vi "Home.TestLauncher.vi"() -> ()   [LabVIEW 2022 SP3, in "Home.lvclass"]
uses:
  Home.lvclass
  Typedefs/Home State--enum.ctl
  <vilib>/JKI/JKI SMO/SMO/Typedefs/SMOState --Enum.ctl
  C:/Program Files (x86)/National Instruments/LabVIEW 2022/vi.lib/JKI/JKI SMO/SMO/SMO.lvclass
  <vilib>/JKI/JKI SMO/SMO/SMO.lvclass/SMO.ctl
  <vilib>/JKI/JKI SMO/SMO/Private/ReftoDVR--SMO.vi
  Home.lvclass/Home.ctl
  <vilib>/JKI/JKI SMO/SMO/SMO.lvclass
  D:/DSUsers/uib01493/000_SD_Card/009_Projects/CIS_580/SReTT_GUI/002_SRC/Home/Home.lvclass
panel:
  out "SMO State":T1
  in  "Embed?":bool=TRUE
  out "UI State":T2
  out "error out":errorcluster
  in  "Stop":bool
  # "SMO.UI_Embedded Test Launcher"
  # "For instructions on how to use the JKI State Machine Objects, examples and video tutorials, visit:\nhttp://jki.net/state-machine-objects/\n\nJKI State Machine Objects™\nhttp://jki.net/state-machine-objects/\nCopyright (C) 2005-2015, JKI <info@jki.net>\nALL RIGHTS RESERVED"
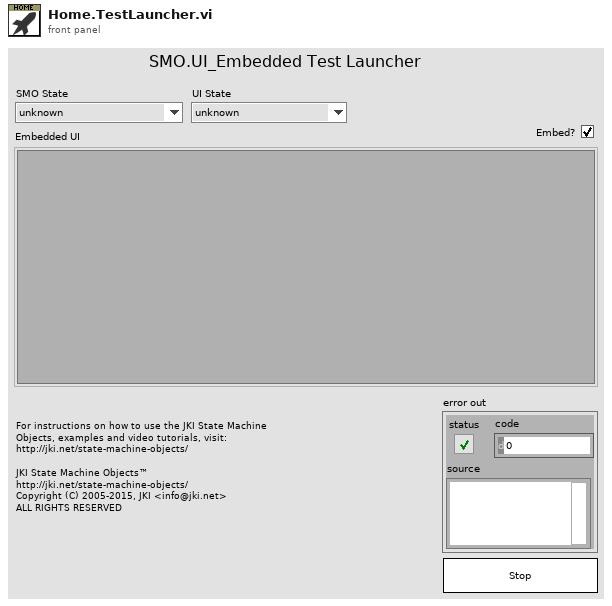
[diagram p1: front panel]
types:
  T1 = typedef "SMO.lvclass/SMOState --Enum.ctl" = enum16{"unknown", "Created", "Started", "Stopped"}
  T2 = typedef "Home.lvclass/Home State--enum.ctl" = enum16{"unknown", "Opened", "Embedded", "Closed"}
  T3 = typedef "SMO.lvclass/Public Events.ctl" = cluster{"Error":refnum<user-event>, "State":refnum<user-event>, "Reserve State":refnum<user-event>}
  T4 = typedef "Home.lvclass/PublicEvents--Cluster.ctl" = cluster{"UI State":refnum<user-event>}
  T5 = cluster{"Event Registration Refnum":refnum<event-registration>}
  T6 = typedef "Home.lvclass/SMO.UI_Embed State--enum.ctl" = enum16{"unknown", "Opened", "Embedded", "Closed"}
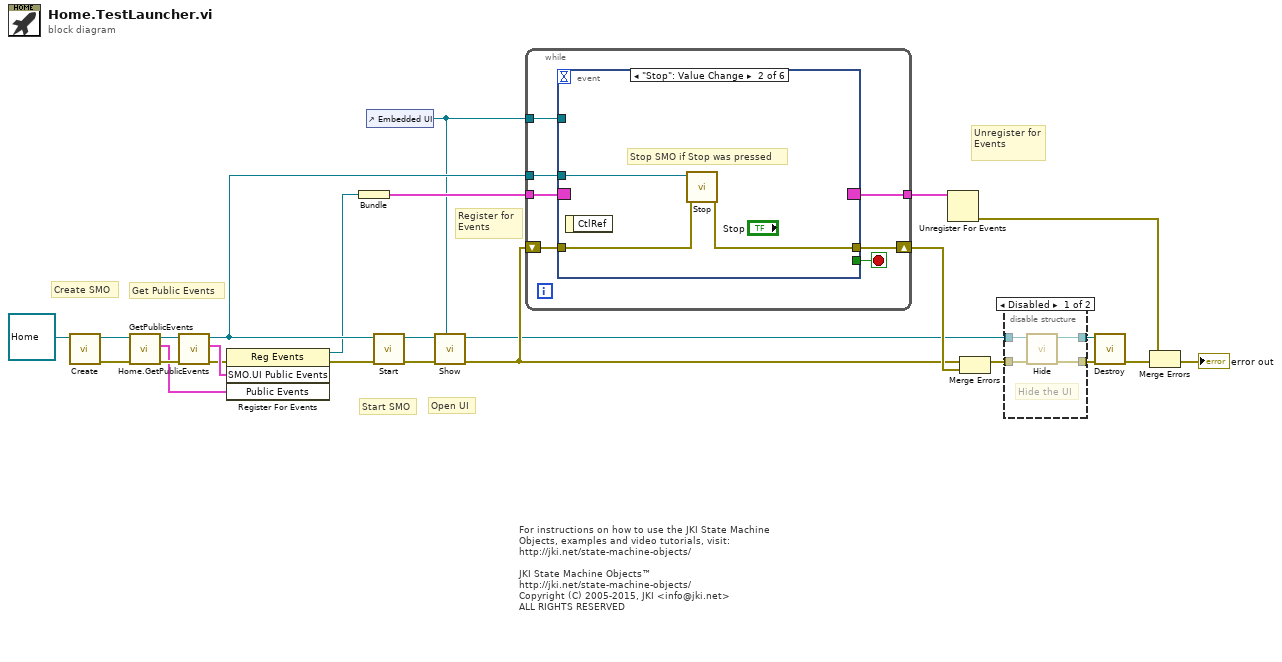
[diagram p0: block diagram]
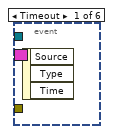
[diagram p3: hidden frame]
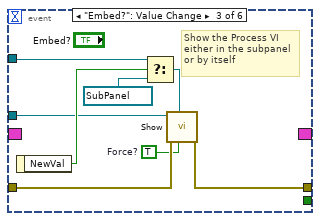
[diagram p4: hidden frame]
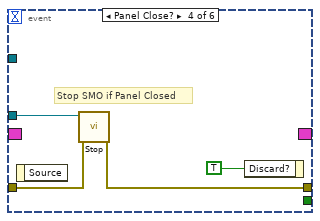
[diagram p5: hidden frame]
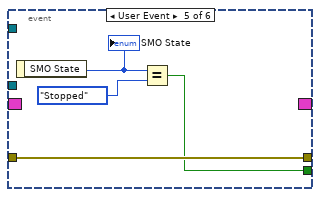
[diagram p6: hidden frame]
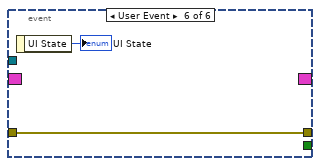
[diagram p7: hidden frame]
diagram:
  # "For instructions on how to use the JKI State Machine Objects, examples and video tutorials, visit:\nhttp://jki.net/state-machine-objects/\n\nJKI State Machine Objects™\nhttp://jki.net/state-machine-objects/\nCopyright (C) 2005-2015, JKI <info@jki.net>\nALL RIGHTS RESERVED"
  # "Get Public Events"
  # "Start SMO"
  # "Create SMO"
  # "Open UI"
  # "Unregister for Events"
  # "Register for Events"
  n1 = call <vilib>:"Create.vi"("SMO"=refnum<class "Home.lvclass"> refnum ("SMO.UI.lvclass")) -> ("error out"=w13:errorcluster, "SMO out"=w11:refnum<class "Home.lvclass">)  [unwired: 8 in, 1 out]
  n2 = call <vilib>:"GetPublicEvents.vi"("error in (no error)"=w13, "SMO"=w11) -> ("error out"=w12:errorcluster, "Public Events"=w9:T3, "SMO out"=w10:refnum<class "Home.lvclass">)  [unwired: 7 in]
  n3 = call "Home.GetPublicEvents.vi"("error in (no error)"=w12, "Home"=w10) -> ("error out"=w15:errorcluster, "SMO.UI Public Events"=w17:T4, "Home out"=w18:refnum<class "Home.lvclass">)  [unwired: 7 in]
  n4 = register-events(error in=w15, w17, w9) -> (reference out=w16:refnum<event-registration>, error out=w14:errorcluster)  [unwired: 1 in]
  n5 = Bundle("Event Registration Refnum"=w16) -> (w24:T5)  [unwired: 1 in]
  n6 = control-ref of="Embedded UI"() -> (w5:refnum<vi>)
  n7 = call <vilib>:"Start.vi"("error in (no error)"=w14, "SMO"=w18) -> ("error out"=w7:errorcluster, "SMO out"=w8:refnum<class "Home.lvclass">)  [unwired: 8 in]
  n8 = call "Show.vi"("Subpanel Ref (empty: open detached)"=w5, "error in (no error)"=w7, "Home"=w8) -> ("error out"=w6:errorcluster, "Home out"=w4:refnum<class "Home.lvclass">)  [unwired: 7 in]
  n9 = while {
    shift-right: [w31] -> w22
    shift-left: w6 -> [w30]
    tunnel: w24 -> [w29]
    tunnel: [w28] -> w25
    tunnel: w18 -> [w27]
    tunnel: w5 -> [w26]
    stop <- w32 stop-if-true
    n10 = event shown="[1] \"Stop\": Value Change" {
      selector: w29 -> [_ _ _ _ _ _]
      dyn-events: [_ _ _ _ _ _] -> w28
      timeout: _ -> [_ _ _ _ _ _]
      tunnel: [_ _ _ _ w48 _] -> w32
      tunnel: w27 -> [_ w33 w38 w47 _ _]
      tunnel: [_ w35 w43 w46 w49 w53] -> w31
      tunnel: w30 -> [_ w34 w37 w45 w49 w53]
      tunnel: w26 -> [_ _ w41 _ _ _]
      event Timeout {
        n11 = event-data() -> ()  [unwired: 1 in, 3 out]
      }
      event "Stop": Value Change {
        # "Stop SMO if Stop was pressed"
        n12 = event-data() -> ()  [unwired: 1 in, 1 out]
        n13 = call <vilib>:"Stop.vi"("error in (no error)"=w34, "SMO"=w33) -> ("error out"=w35:errorcluster)  [unwired: 8 in, 1 out]
      }
      event "Embed?": Value Change {
        w36 = TRUE  # Force?
        # "Show the Process VI\neither in the subpanel\nor by itself"
        n14 = event-data() -> ("NewVal"=w42:bool)  [unwired: 1 in]
        n15 = Select(t=w41, s=w42, f=refnum<vi> refnum) -> (s? t:f=w40:refnum<vi>)
        n16 = call "Show.vi"("Force? (true)"=w36, "Subpanel Ref (empty: open detached)"=w40, "error in (no error)"=w37, "Home"=w38) -> ("error out"=w43:errorcluster)  [unwired: 6 in, 1 out]
      }
      event Panel Close? {
        # "Stop SMO if Panel Closed"
        n17 = event-data() -> ()  [unwired: 1 in, 1 out]
        n18 = call <vilib>:"Stop.vi"("error in (no error)"=w45, "SMO"=w47) -> ("error out"=w46:errorcluster)  [unwired: 8 in, 1 out]
        n19 = event-data("Discard?"=TRUE ("OK")) -> ()  [unwired: 1 in, 1 out]
      }
      event User Event {
        n20 = event-data() -> ("SMO State"=w51:T1)  [unwired: 1 in]
        "SMO State" <- w51
        n21 = Equal?(x=w51, y=SMOState_--Enum."Stopped") -> (x = y?=w48:bool)
      }
      event User Event {
        n22 = event-data() -> ("UI State"=→"UI State":T6)  [unwired: 1 in]
      }
    }
  }
  n23 = Unregister For Events(event registration refnum=w25) -> (error out=w21:errorcluster)  [unwired: 1 in]
  n24 = Merge Errors(w6, w22) -> (w2:errorcluster)
  n25 = disable-structure shown="Disabled" {
    disable-tunnel: w4 -> [w57 w59]
    disable-tunnel: [w56 w59] -> w3
    disable-tunnel: w2 -> [w55 w58]
    disable-tunnel: [w54 w58] -> w1
    frame Disabled {
      # "Hide the UI"
      n26 = call "Hide.vi"("error in (no error)"=w55, "Home"=w57) -> ("error out"=w54:errorcluster, "Home out"=w56:refnum<class "Home.lvclass">)  [unwired: 8 in]
    }
    frame Enabled {
    }
  }
  n27 = call <vilib>:"Destroy.vi"("error in (no error)"=w1, "SMO"=w3) -> ("error out"=w19:errorcluster)  [unwired: 9 in]
  n28 = Merge Errors(w21, w19) -> (→"error out":errorcluster)
